vi "pp.vi"(0 "Waveform":waveform(dbl), 1 "mean/sample max":dbl, 2 "std dev max":dbl, 5 "SAVE?":bool, 7 "prev std dev":dbl, 9 "prev mean":dbl) -> (4 "out":bool, 6 "mean":bool, 8 "std dev":bool, 10 "mean":dbl format="%0.2f", 13 "std dev/semple":dbl, 14 "mean/sample":dbl, 15 "standard deviation":dbl format="%0.2f")   [LabVIEW 2017]
uses:
  <vilib>/Analysis/NI_AALBase.lvlib
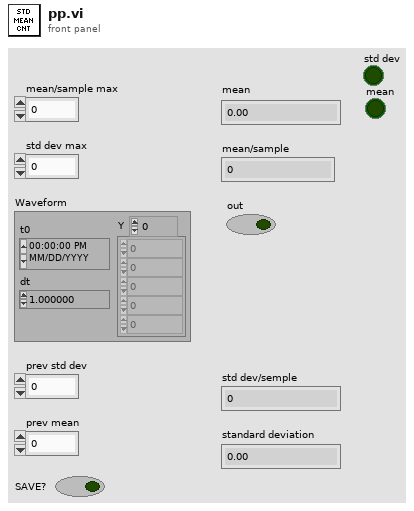
[diagram p1: front panel]
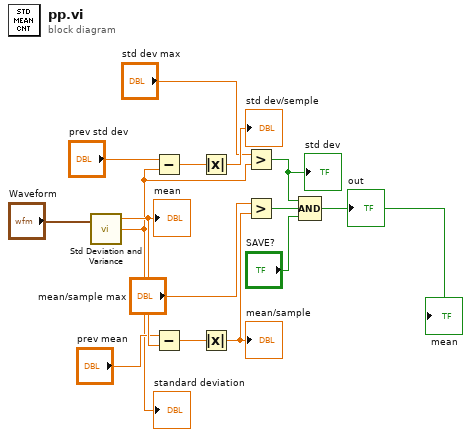
[diagram p0: block diagram]
diagram:
  n1 = call <vilib>:"Std Deviation and Variance.vi"("X"="Waveform") -> ("mean"=w8:dbl, "standard deviation"=w1:dbl)  [unwired: 1 in, 1 out]
  "standard deviation" <- w1
  "mean" <- w8
  n2 = Subtract(x="prev std dev", y=w1) -> (x-y=w4:dbl)
  n3 = Subtract(x="prev mean", y=w8) -> (x-y=w6:dbl)
  n4 = Absolute Value(x=w4) -> (abs(x)=→"std dev/semple":dbl)
  n5 = Absolute Value(x=w6) -> (abs(x)=w13:dbl)
  "mean/sample" <- w13
  n6 = Greater?(x="std dev max", y=w1) -> (0:w12:bool)
  "std dev" <- w12
  n7 = Greater?(x="mean/sample max", y=w13) -> (0:w11:bool)
  "mean" <- w11
  n8 = Compound Arithmetic op=AND(w12, w11, "SAVE?") -> (→"out":bool)
